vi "Get ItemName.vi"(7 "error in (no error)":errorcluster, 8 "Active Cell":cluster{"Row":i32, "Column":i32}, 10 "Multicolumn Listbox":refnum<vi>) -> (0 "error out":errorcluster, 3 "String":string)   [LabVIEW 2012]
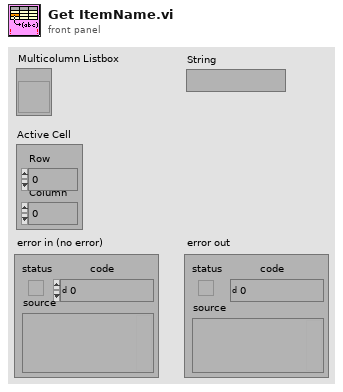
[diagram p1: front panel]
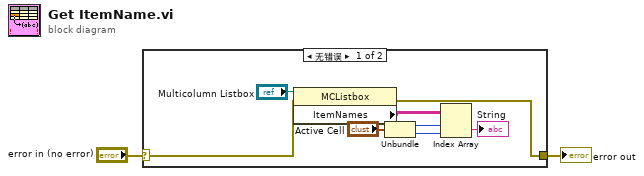
[diagram p0: block diagram]
diagram:
  n1 = case shown="无错误" "error in (no error)" {
    selector: "error in (no error)" -> [w4 w11]
    tunnel: [w3 w11] -> w1
    frame No Error {
      n2 = property class="MCListbox"(reference="Multicolumn Listbox", error in=w4) -> (error out=w3:errorcluster, "ItemNames"=w7:string[][])  [unwired: 1 out]
      n3 = Unbundle("Active Cell") -> ("Row"=w8:i32, "Column"=w9:i32)
      n4 = Index Array(array=w7, index (row)=w8, index (col)=w9) -> (element=→"String":string)
    }
    frame Error {
    }
  }
  "error out" <- w1
